vi "GFITS_SetHdrVar.vi"(8 "error in (no error)":errorcluster, 9 "data":string, 10 "args":string) -> (0 "error out":errorcluster, 2 "response":string)   [LabVIEW 2016]
uses:
  DBSHAND/private/vis/DatabaseHand_Element_Set(string).vi
  DBSHAND/private/vis/DatabaseHand_Element_Set(double).vi
  DBSHAND/private/vis/DatabaseHand_Element_Set(I32).vi
  DBSHAND/private/vis/DatabaseHand_Element_Set(U32).vi
  DBSHAND/private/vis/DatabaseHand_Element_Set(I16).vi
  DBSHAND/private/vis/DatabaseHand_Element_Set(U16).vi
  DBSHAND/private/vis/DatabaseHand_Element_Set(2DArr).vi
  DBSHAND/private/vis/DatabaseHand_Element_Set(1DArr).vi
  DBSHAND/private/vis/DatabaseHand_Element_Set(bool).vi
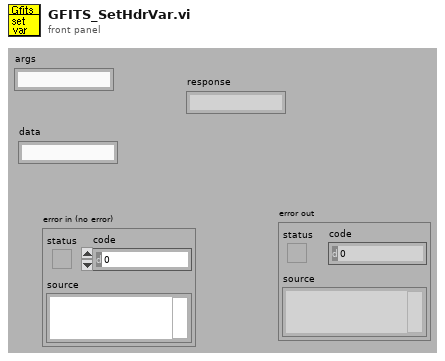
[diagram p1: front panel]
types:
  T1 = typedef "DatabaseHand_RefNum.ctl" = refnum<vi>
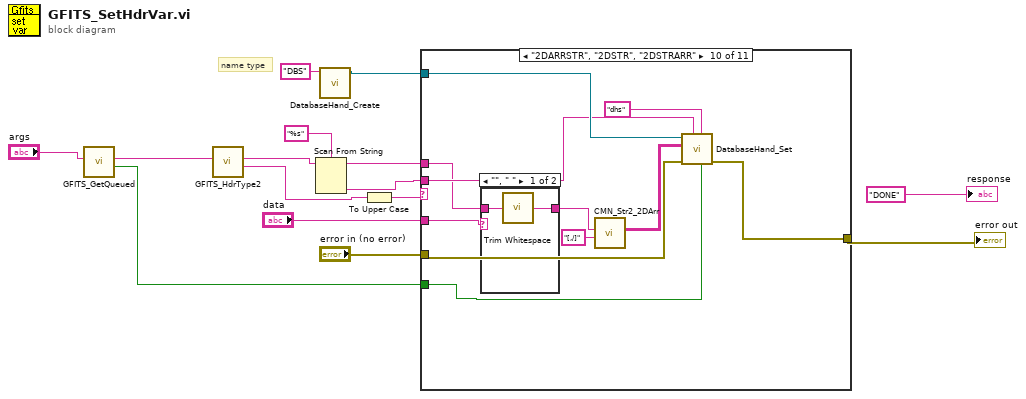
[diagram p0: block diagram]
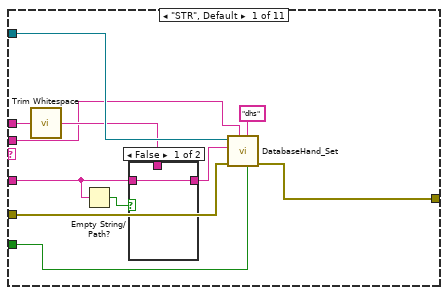
[diagram p2: hidden frame]
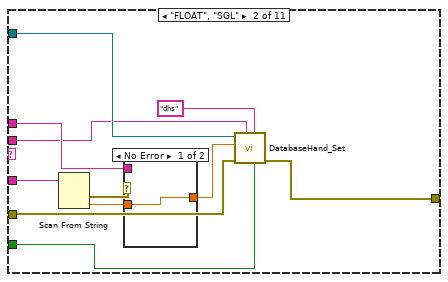
[diagram p4: hidden frame]
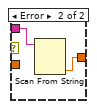
[diagram p5: hidden frame]
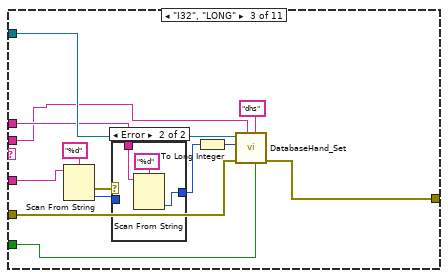
[diagram p6: hidden frame]
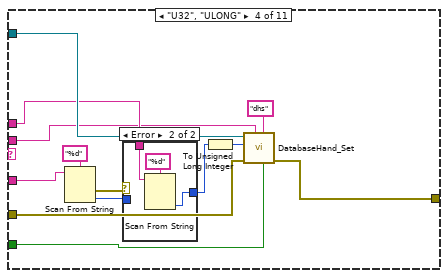
[diagram p8: hidden frame]
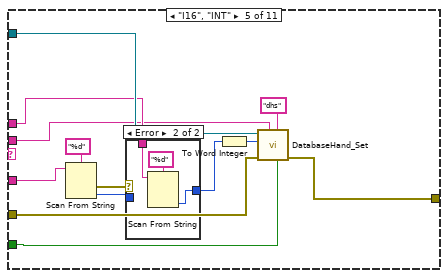
[diagram p10: hidden frame]
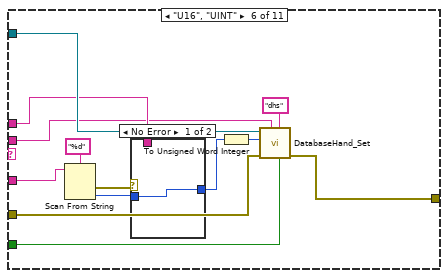
[diagram p12: hidden frame]
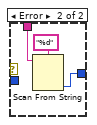
[diagram p13: hidden frame]
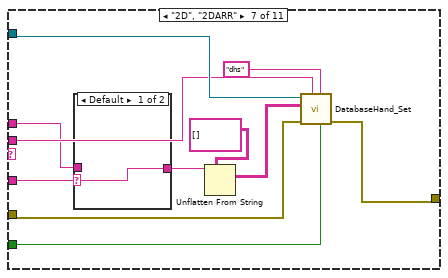
[diagram p14: hidden frame]
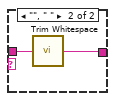
[diagram p15: hidden frame]
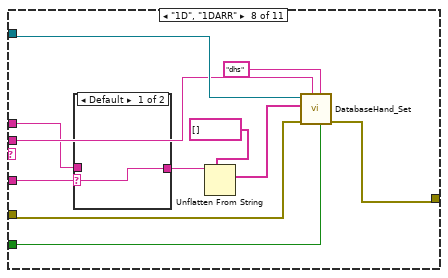
[diagram p16: hidden frame]
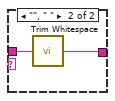
[diagram p17: hidden frame]
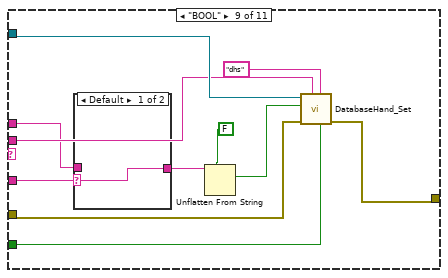
[diagram p18: hidden frame]
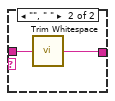
[diagram p19: hidden frame]
diagram:
  # "name type"
  n1 = call "GFITS_GetQueued.vi"("input"="args") -> ("queued?"=w1:bool, "output"=w2:string)  [unwired: 9 out]
  n2 = call "GFITS_HdrType2.vi"("keyval"=w2) -> ("type"=w9:string, "keyval out"=w10:string)  [unwired: 9 out]
  n3 = Scan From String(format string="%s", input string=w10) -> (remaining string=w8:string, output 1=w13:string)  [unwired: 2 in, 3 out]
  n4 = call "DatabaseHand_Create.vi"("Name"="DBS") -> ("Database RefNum out"=w7:T1)  [unwired: 1 in, 9 out]
  n5 = To Upper Case(1:w9) -> (0:w11:string)
  n6 = case shown="\"2DARRSTR\", \"2DSTR\", \"2DSTRARR\"" w11 {
    tunnel: w7 -> [w25 w38 w54 w71 w88 w105 w121 w135 w149 w163 _]
    tunnel: "data" -> [w21 w35 w51 w68 w85 w102 w111 w126 w140 w157 _]
    tunnel: w13 -> [w17 w30 w44 w61 w78 w95 w120 w134 w148 w156 _]
    tunnel: "error in (no error)" -> [w23 w36 w52 w69 w86 w103 w116 w130 w144 w161 w171]
    tunnel: [w24 w37 w53 w70 w87 w104 w115 w129 w143 w160 w167] -> w5
    tunnel: w8 -> [w19 w31 w45 w63 w80 w97 w114 w128 w142 w153 _]
    tunnel: w1 -> [w16 w29 w43 w60 w77 w94 w112 w125 w139 w154 _]
    frame "STR", Default {
      n7 = call <vilib>:"Trim Whitespace.vi"("string"=w19) -> ("trimmed string"=w18:string)  [unwired: 1 in]
      n8 = Empty String/Path?(string/path=w21) -> (empty?=w22:bool)
      n9 = case shown="False" w22 {
        tunnel: w21 -> [w27 _]
        tunnel: [w27 w28] -> w20
        tunnel: w18 -> [_ w28]
        frame False {
        }
        frame True {
        }
      }
      n10 = call-poly "DatabaseHand_Set.vi"("enqueue? (F)"=w16, "group"="dhs", "name"=w17, "error in (no error)"=w23, "value"=w20, "Database RefNum in"=w25) -> ("error out"=w24:errorcluster)  [unwired: 2 in, 3 out]
    }
    frame "FLOAT", "SGL" {
      n11 = Scan From String(input string=w35) -> (error out=w34:errorcluster, output 1=w33:dbl)  [unwired: 3 in, 3 out]
      n12 = case shown="No Error" w34 {
        tunnel: w33 -> [w40 _]
        tunnel: [w40 w41] -> w32
        tunnel: w31 -> [_ w42]
        frame No Error {
        }
        frame Error {
          n13 = Scan From String(input string=w42) -> (output 1=w41:dbl)  [unwired: 3 in, 4 out]
        }
      }
      n14 = call-poly "DatabaseHand_Set.vi"("enqueue? (F)"=w29, "group"="dhs", "name"=w30, "error in (no error)"=w36, "value"=w32, "Database RefNum in"=w38) -> ("error out"=w37:errorcluster)  [unwired: 2 in, 3 out]
    }
    frame "I32", "LONG" {
      n15 = Scan From String(format string="%d", input string=w51) -> (error out=w46:errorcluster, output 1=w48:i32)  [unwired: 2 in, 3 out]
      n16 = case shown="Error" w46 {
        tunnel: w48 -> [w56 _]
        tunnel: [w56 w59] -> w47
        tunnel: w45 -> [_ w57]
        frame No Error {
        }
        frame Error {
          n17 = Scan From String(format string="%d", input string=w57) -> (output 1=w59:i32)  [unwired: 2 in, 4 out]
        }
      }
      n18 = To Long Integer(number=w47) -> (32bit integer=w49:i32)
      n19 = call-poly "DatabaseHand_Set.vi"("enqueue? (F)"=w43, "group"="dhs", "name"=w44, "error in (no error)"=w52, "value"=w49, "Database RefNum in"=w54) -> ("error out"=w53:errorcluster)  [unwired: 2 in, 3 out]
    }
    frame "U32", "ULONG" {
      n20 = Scan From String(format string="%d", input string=w68) -> (error out=w62:errorcluster, output 1=w65:i32)  [unwired: 2 in, 3 out]
      n21 = case shown="Error" w62 {
        tunnel: w65 -> [w73 _]
        tunnel: [w73 w76] -> w64
        tunnel: w63 -> [_ w74]
        frame No Error {
        }
        frame Error {
          n22 = Scan From String(format string="%d", input string=w74) -> (output 1=w76:i32)  [unwired: 2 in, 4 out]
        }
      }
      n23 = To Unsigned Long Integer(number=w64) -> (unsigned 32bit integer=w66:u32)
      n24 = call-poly "DatabaseHand_Set.vi"("enqueue? (F)"=w60, "group"="dhs", "name"=w61, "error in (no error)"=w69, "value"=w66, "Database RefNum in"=w71) -> ("error out"=w70:errorcluster)  [unwired: 2 in, 3 out]
    }
    frame "I16", "INT" {
      n25 = Scan From String(format string="%d", input string=w85) -> (error out=w79:errorcluster, output 1=w82:i32)  [unwired: 2 in, 3 out]
      n26 = case shown="Error" w79 {
        tunnel: w82 -> [w90 _]
        tunnel: [w90 w93] -> w81
        tunnel: w80 -> [_ w91]
        frame No Error {
        }
        frame Error {
          n27 = Scan From String(format string="%d", input string=w91) -> (output 1=w93:i32)  [unwired: 2 in, 4 out]
        }
      }
      n28 = To Word Integer(number=w81) -> (16bit integer=w83:i16)
      n29 = call-poly "DatabaseHand_Set.vi"("enqueue? (F)"=w77, "group"="dhs", "name"=w78, "error in (no error)"=w86, "value"=w83, "Database RefNum in"=w88) -> ("error out"=w87:errorcluster)  [unwired: 2 in, 3 out]
    }
    frame "U16", "UINT" {
      n30 = Scan From String(format string="%d", input string=w102) -> (error out=w96:errorcluster, output 1=w99:i32)  [unwired: 2 in, 3 out]
      n31 = case shown="No Error" w96 {
        tunnel: w99 -> [w107 _]
        tunnel: [w107 w110] -> w98
        tunnel: w97 -> [_ w108]
        frame No Error {
        }
        frame Error {
          n32 = Scan From String(format string="%d", input string=w108) -> (output 1=w110:i32)  [unwired: 2 in, 4 out]
        }
      }
      n33 = To Unsigned Word Integer(number=w98) -> (unsigned 16bit integer=w100:u16)
      n34 = call-poly "DatabaseHand_Set.vi"("enqueue? (F)"=w94, "group"="dhs", "name"=w95, "error in (no error)"=w103, "value"=w100, "Database RefNum in"=w105) -> ("error out"=w104:errorcluster)  [unwired: 2 in, 3 out]
    }
    frame "2D", "2DARR" {
      n35 = case shown="Default" w111 {
        selector: w111 -> [w122 _]
        tunnel: w114 -> [_ w124]
        tunnel: [w122 w123] -> w113
        frame Default {
        }
        frame "", " " {
          n36 = call <vilib>:"Trim Whitespace.vi"("string"=w124) -> ("trimmed string"=w123:string)  [unwired: 1 in]
        }
      }
      n37 = Unflatten From String(type=string[][] [], binary string=w113) -> (value=w117:string[][])  [unwired: 1 in, 4 out]
      n38 = call-poly "DatabaseHand_Set.vi"("enqueue? (F)"=w112, "group"="dhs", "name"=w120, "error in (no error)"=w116, "value"=w117, "Database RefNum in"=w121) -> ("error out"=w115:errorcluster)  [unwired: 2 in, 3 out]
    }
    frame "1D", "1DARR" {
      n39 = case shown="Default" w126 {
        selector: w126 -> [w136 _]
        tunnel: w128 -> [_ w138]
        tunnel: [w136 w137] -> w127
        frame Default {
        }
        frame "", " " {
          n40 = call <vilib>:"Trim Whitespace.vi"("string"=w138) -> ("trimmed string"=w137:string)  [unwired: 1 in]
        }
      }
      n41 = Unflatten From String(type=string[] [], binary string=w127) -> (value=w131:string[])  [unwired: 1 in, 4 out]
      n42 = call-poly "DatabaseHand_Set.vi"("enqueue? (F)"=w125, "group"="dhs", "name"=w134, "error in (no error)"=w130, "value"=w131, "Database RefNum in"=w135) -> ("error out"=w129:errorcluster)  [unwired: 3 in, 2 out]
    }
    frame "BOOL" {
      n43 = case shown="Default" w140 {
        selector: w140 -> [w150 _]
        tunnel: w142 -> [_ w152]
        tunnel: [w150 w151] -> w141
        frame Default {
        }
        frame "", " " {
          n44 = call <vilib>:"Trim Whitespace.vi"("string"=w152) -> ("trimmed string"=w151:string)  [unwired: 1 in]
        }
      }
      n45 = Unflatten From String(type=FALSE, binary string=w141) -> (value=w145:bool)  [unwired: 1 in, 4 out]
      n46 = call-poly "DatabaseHand_Set.vi"("enqueue? (F)"=w139, "group"="dhs", "name"=w148, "error in (no error)"=w144, "value"=w145, "Database RefNum in"=w149) -> ("error out"=w143:errorcluster)  [unwired: 2 in, 3 out]
    }
    frame "2DARRSTR", "2DSTR", "2DSTRARR" {
      n47 = case shown="\"\", \" \"" w157 {
        selector: w157 -> [_ w166]
        tunnel: w153 -> [w165 _]
        tunnel: [w164 w166] -> w155
        frame "", " " {
          n48 = call <vilib>:"Trim Whitespace.vi"("string"=w165) -> ("trimmed string"=w164:string)  [unwired: 1 in]
        }
        frame Default {
        }
      }
      n49 = call "CMN_Str2_2DArr.vi"("col separator"="[,/]", "multi line string in"=w155) -> ("array out"=w159:string[][])  [unwired: 9 out]
      n50 = call-poly "DatabaseHand_Set.vi"("enqueue? (F)"=w154, "group"="dhs", "name"=w156, "error in (no error)"=w161, "value"=w159, "Database RefNum in"=w163) -> ("error out"=w160:errorcluster)  [unwired: 2 in, 3 out]
    }
    frame "", " " {
      n51 = Bundle By Name(cluster=w171, "status"=TRUE, "code"=-22, "source"="ERROR invalid variable name") -> (w167:errorcluster)
    }
  }
  "error out" <- w5
  "response" <- "DONE" ("ok response")
